vi "All Joystick Values.vi"() -> ()   [LabVIEW 2013]
uses:
  <vilib>/Rock Robotics/WPI/Joystick/WPI_JoystickButtonState.ctl
  <vilib>/Rock Robotics/WPI/Joystick/WPI_JoystickAxis.ctl
  <vilib>/Rock Robotics/WPI/Joystick/WPI_JoystickGetSetRefNum.vi
panel:
  out "Value":dbl
  in  "Axis":T1
  out "RAW Buttons":T2
  out "RAW Axes":T3
  out "Buttons":T2
  out "Axes":T4
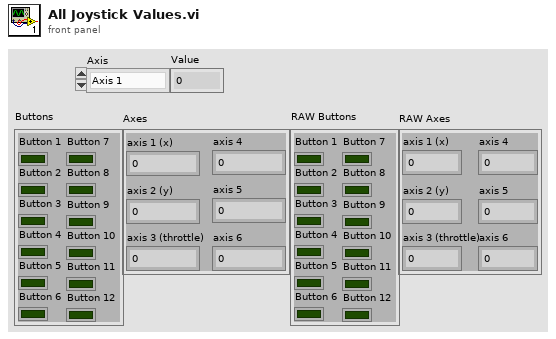
[diagram p1: front panel]
types:
  T1 = typedef "WPI_JoystickAxis.ctl" = enum16{"Axis 1", "Axis 2", "Axis 3", "Axis 4", "Axis 5", "Axis 6"}
  T2 = typedef "WPI_JoystickButtonState.ctl" = cluster{"Button 1":bool, "Button 2":bool, "Button 3":bool, "Button 4":bool, "Button 5":bool, "Button 6":bool, "Button 7":bool, "Button 8":bool, "Button 9":bool, "Button 10":bool, "Button 11":bool, "Button 12":bool}
  T3 = cluster{"axis 1 (x)":i8, "axis 2 (y)":i8, "axis 3 (throttle)":i8, "axis 4":i8, "axis 5":i8, "axis 6":i8}
  T4 = cluster{"axis 1 (x)":dbl, "axis 2 (y)":dbl, "axis 3 (throttle)":dbl, "axis 4":dbl, "axis 5":dbl, "axis 6":dbl}
  T5 = typedef "WPI_JoystickDevRef.ctl" = cluster{"Device":T6}
  T6 = typedef "WPI_JoystickDeviceEnum.ctl" = enum16{"USB 1", "USB 2", "USB 3", "USB 4", "Kinect 1", "Kinect 2"}
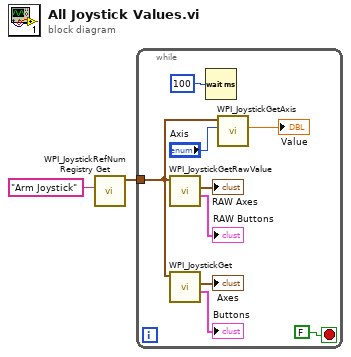
[diagram p0: block diagram]
diagram:
  n1 = call <vilib>:"WPI_JoystickRefNum Registry Get.vi"("refnum name"="Arm Joystick") -> ("JoystickDevRef"=w2:T5)  [unwired: 9 in, 1 out]
  n2 = while {
    tunnel: w2 -> [w5]
    stop <- FALSE stop-if-true
    n3 = call <vilib>:"WPI_JoystickGetRawValue.vi"("JoystickDevRef"=w5) -> ("Buttons"=→"RAW Buttons":T2, "Axes"=→"RAW Axes":T3)  [unwired: 8 in, 1 out]
    n4 = call <vilib>:"WPI_JoystickGet.vi"("JoystickDevRef"=w5) -> ("Buttons"=→"Buttons":T2, "Axes"=→"Axes":T4)  [unwired: 4 in, 1 out]
    n5 = Wait (ms)(milliseconds to wait=u32 100) -> ()  [unwired: 1 out]
    n6 = call <vilib>:"WPI_JoystickGetAxis.vi"("Axis"="Axis", "JoystickDevRef"=w5) -> ("Value"=→"Value":dbl)  [unwired: 8 in, 1 out]
  }
